vi "Read Operator.vi"(8 "error in (no error)":errorcluster, 11 "Engine in":refnum<class "Engine.lvclass">) -> (0 "error out":errorcluster, 2 "Operator":string, 3 "Engine out":refnum<class "Engine.lvclass">)   [LabVIEW 2023, in "Engine.lvlib" / "Engine.lvclass"]
uses:
  Library/Engine.lvclass
  Library/Engine.lvclass/Engine.ctl
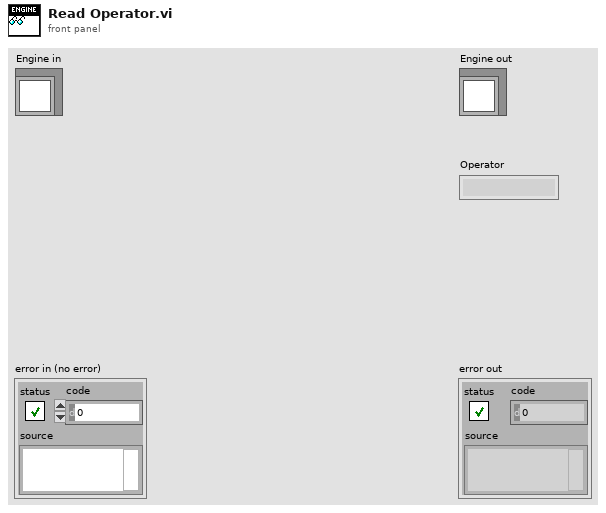
[diagram p1: front panel]
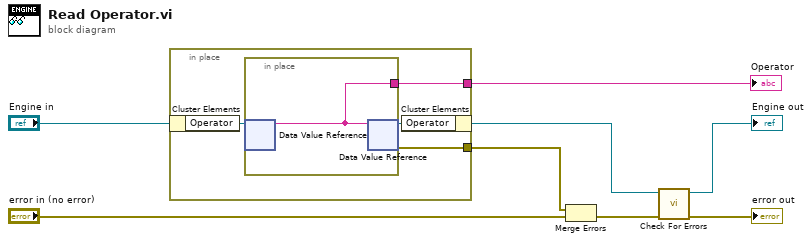
[diagram p0: block diagram]
diagram:
  n1 = in-place {
    in-place-border: [w10] -> w7
    in-place-border: [w9] -> w1
    n2 = in-place-cluster #1("Engine in") -> ("Operator"=w12:refnum<data-value>)
    n3 = in-place {
      in-place-border: [w13] -> w9
      n4 = in-place-dvr #2(w12) -> (w13:string)  [unwired: 1 out]
      n5 = in-place-dvr #2(w13) -> (w11:refnum<data-value>, w10:errorcluster)
    }
    n6 = in-place-cluster #1("Operator"=w11) -> (w3:refnum<class "Engine.lvclass">)
  }
  "Operator" <- w1
  n7 = Merge Errors(w7, "error in (no error)") -> (w5:errorcluster)
  n8 = call "Check For Errors.vi"("error in"=w5, "Engine in"=w3) -> ("error out"=→"error out":errorcluster, "Engine out"=→"Engine out":refnum<class "Engine.lvclass">)  [unwired: 8 in]
